vi "motor calibration.vi"() -> ()   [LabVIEW 2015]
panel:
  in  "stop":bool
  in  "Speed":dbl min=0.0 max=1.0 step=0.0005 format="%#_13g"
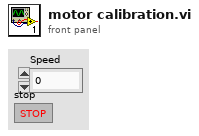
[diagram p1: front panel]
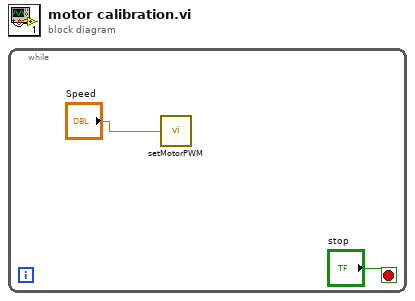
[diagram p0: block diagram]
diagram:
  n1 = while {
    stop <- "stop" stop-if-true
    n2 = call "setMotorPWM.vi"("Numeric"="Speed") -> ()
  }
